vi "PR Current Trigger Delay.vi"() -> (0 "TriggerDelay":i32)   [LabVIEW 2022 SP3, in "BS6006PRPLUS.lvlib"]
doc: "The function gets the trigger delay for acquiring signals.\n\nextern \"C\" BS6006PRPLUS_API int __cdecl PR_CurrentTriggerDelay();"
uses:
  BS6006PRPLUS.lvlib
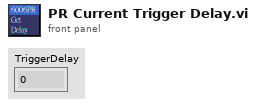
[diagram p1: front panel]
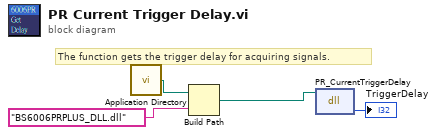
[diagram p0: block diagram]
diagram:
  # "The function gets the trigger delay for acquiring signals."
  n1 = call <vilib>:"Application Directory.vi"() -> ("Application Directory"=w3:path)
  n2 = Build Path(base path=w3, name or relative path="BS6006PRPLUS_DLL.dll") -> (appended path=w1:path)
  n3 = dll-call lib="E:/Broadsound_Program/PulserReceiver/6006PR PLUS/API/DLL/LabVIEW 15/VIs/BS6006PRPLUS_DLL.dlls" fn="PR_CurrentTriggerDelay"(path in=w1) -> ("return type"=→"TriggerDelay":i32)  [unwired: 2 in, 2 out]
